vi "Performance test.vi"() -> ()   [LabVIEW 2009]
panel:
  in  "deviceId":i32
  in  "Path to LUT file":path=path "C:/BLINK_PCIe/LUT_Files/linear.lut"
  out "XY Graph":cluster{i32[], dbl[]}(graph)={[1, 2], [4.621621621621622, 5.528528528528528]}
  out "Last number of spots":i32=1
  out "Last execution time":dbl=5.528528528528528
  in  "alpha RPC":sgl=1.0
  in  "Number of spotsmax":i32=100
  in  "Number of spots min":i32=1
  in  "TrueFrame":i32=3
  in  "Number of \ntime to execute":i32=100
  in  "stop program":bool
  out "Generated Hologram":u8[][](graph)
  in  "Method":i32(ring)=1 items=["Lenses & Gratings (3D)", "Gerschberg-Saxton Fresnel (3D)", "Gerschberg-Saxton FFT (2D)"]
  in  "N_iterations":i32=10
  in  "SLM enabled":bool
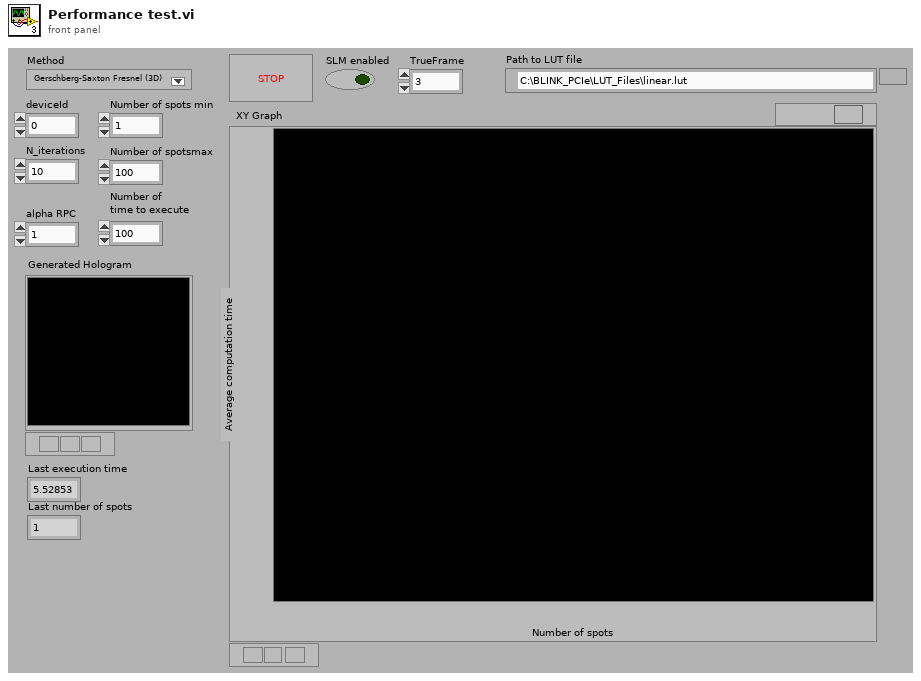
[diagram p1: front panel]
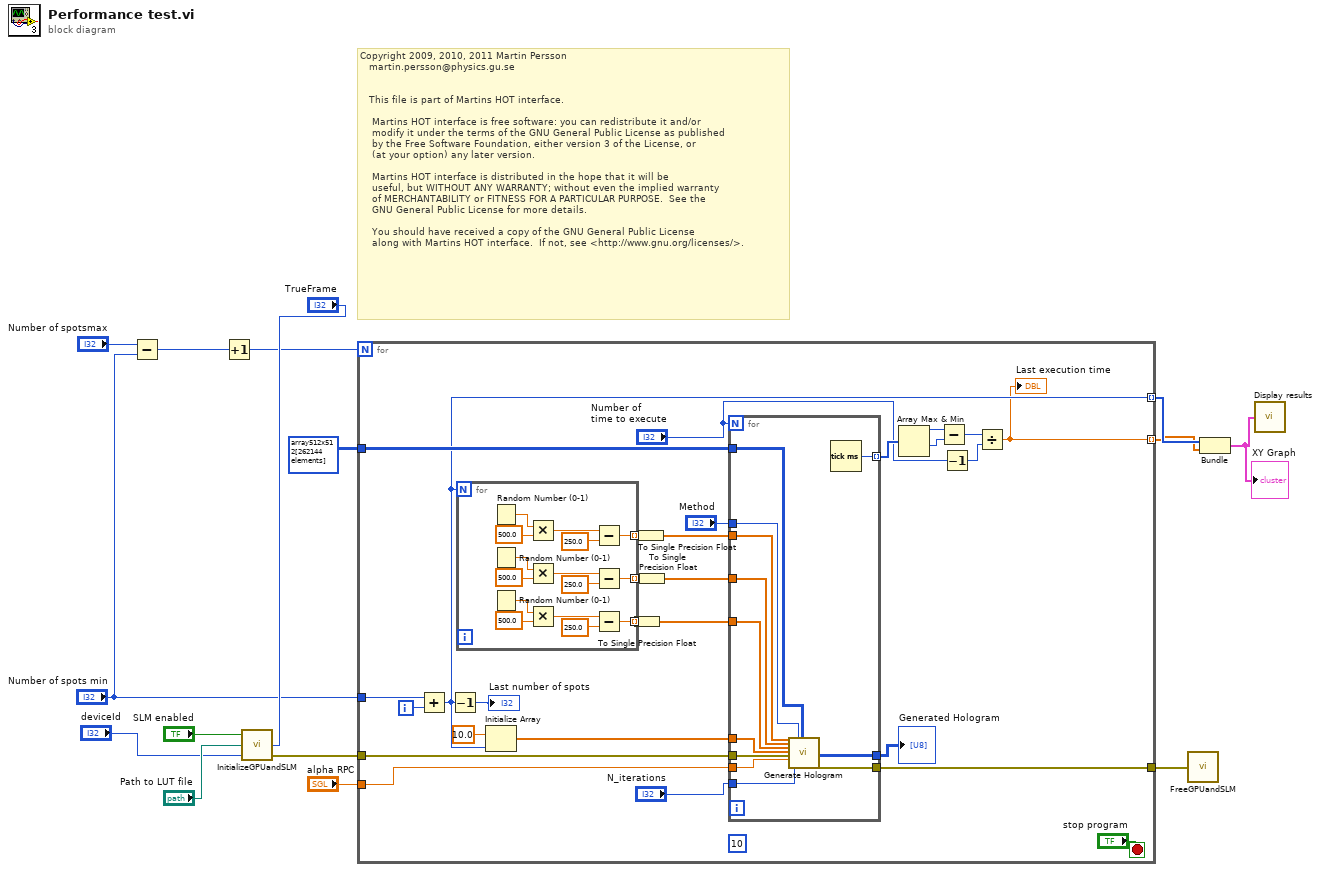
[diagram p0: block diagram]
diagram:
  # "Copyright 2009, 2010, 2011 Martin Persson \n   martin.persson@physics.gu.se\n\n\n   This file is part of Martins HOT interface.\n\n    Martins HOT interface is free software: you can redistribute it and/or \n    modify it under the terms of the GNU General Public License as published \n    by the Free Software Foundation, either version 3 of the License, or\n    (at your option) any later version.\n\n    Martins HOT interface is distributed in the hope that it will be \n    useful, but WITHOUT ANY WARRANTY; without even the implied warranty\n    of MERCHANTABILITY or FITNESS FOR A PARTICULAR PURPOSE.  See the\n    GNU General Public License for more details.\n\n    You should have received a copy of the GNU General Public License\n    along with Martins HOT interface.  If not, see <http://www.gnu.org/licenses/>."
  n1 = Subtract(x="Number of spotsmax", y="Number of spots min") -> (x-y=w10:i32)
  n2 = Increment(x=w10) -> (x+1=w8:i32)
  n3 = call "InitializeGPUandSLM.vi"("TrueFrame"="TrueFrame", "deviceId"="deviceId", "Path to LUT file"="Path to LUT file", "SLM enabled"="SLM enabled") -> ("CUDA/SLM error"=w14:errorcluster)  [unwired: 1 out]
  n4 = for {
    N: w8 -> [_]
    tunnel: w14 -> [w42]
    tunnel: [w39] -> w13
    tunnel: u8[][] array512x512[262144 elements] ("Default") -> [w37]
    tunnel: "Number of spots min" -> [w29]
    tunnel: [w21] -> w3 mode=indexing
    tunnel: [w22] -> w4 mode=indexing
    tunnel: "alpha RPC" -> [w24]
    i -> [w28]
    stop <- "stop program" stop-if-true
    (unwired) 10 ("element")
    n5 = Add(x=w29, y=w28) -> (x+y=w22:i32)
    n6 = Decrement(x=w22) -> (x-1=→"Last number of spots":i32)
    n7 = for {
      N: w22 -> [_]
      tunnel: [w46] -> w27 mode=indexing
      tunnel: [w45] -> w26 mode=indexing
      tunnel: [w44] -> w25 mode=indexing
      n8 = Random Number (0-1)() -> (number: 0 to 1=w57:dbl)
      n9 = Random Number (0-1)() -> (number: 0 to 1=w50:dbl)
      n10 = Random Number (0-1)() -> (number: 0 to 1=w43:dbl)
      n11 = Multiply(x=w57, y=500.0) -> (x*y=w55:dbl)
      n12 = Multiply(x=w50, y=500.0) -> (x*y=w52:dbl)
      n13 = Multiply(x=w43, y=500.0) -> (x*y=w48:dbl)
      n14 = Subtract(x=w55, y=250.0) -> (x-y=w46:dbl)
      n15 = Subtract(x=w52, y=250.0) -> (x-y=w45:dbl)
      n16 = Subtract(x=w48, y=250.0) -> (x-y=w44:dbl)
    }
    n17 = Initialize Array(sgl 10.0 ("element"), w22) -> (w35:sgl[])
    n18 = To Single Precision Float(number=w25) -> (single precision float=w17:sgl[])
    n19 = To Single Precision Float(number=w27) -> (single precision float=w19:sgl[])
    n20 = To Single Precision Float(number=w26) -> (single precision float=w18:sgl[])
    n21 = for {
      N: "Number of \ntime to execute" -> [_]
      tunnel: w42 -> [w69]
      tunnel: "N_iterations" -> [w68]
      tunnel: w18 -> [w67]
      tunnel: w17 -> [w66]
      tunnel: "Method" -> [w65]
      tunnel: [w64] -> w39
      tunnel: [w63] -> w38
      tunnel: w37 -> [w62]
      tunnel: w19 -> [w61]
      tunnel: w35 -> [w60]
      tunnel: [w59] -> w34 mode=indexing
      tunnel: w24 -> [w58]
      n22 = call "Generate Hologram.vi"("x"=w61, "y"=w67, "z"=w66, "spot_intensities"=w60, "CUDA/SLM error in"=w69, "alpha RPC"=w58, "N_iterations"=w68, "method"=w65, "CGH in"=w62) -> ("CGH out"=w63:u8[][], "CUDA/SLM error out"=w64:errorcluster)  [unwired: 16 in, 1 out]
      n23 = Tick Count (ms)() -> (millisecond timer value=w59:u32)
    }
    "Generated Hologram" <- w38
    n24 = Array Max & Min(array=w34) -> (max value=w33:u32, min value=w32:u32)  [unwired: 2 out]
    n25 = Subtract(x=w33, y=w32) -> (x-y=w31:u32)
    n26 = Decrement(x="Number of \ntime to execute") -> (x-1=w20:i32)
    n27 = Divide(x=w31, y=w20) -> (x/y=w21:dbl)
    "Last execution time" <- w21
  }
  n28 = call "FreeGPUandSLM.vi"("error in"=w13) -> ()  [unwired: 2 out]
  n29 = Bundle(w4, w3) -> (w2:cluster{i32[], dbl[]})  [unwired: 1 in]
  "XY Graph" <- w2
  n30 = call "Display results.vi"("Cluster"=w2) -> ()
